vi "Create Instance.vi"() -> (2 "LT_UpgradeFlash":refnum<class "LT_UpgradeFlash.lvclass">)   [LabVIEW 2017, in "LT_UpgradeFlash.lvclass"]
uses:
  LT_UpgradeFlash.lvclass
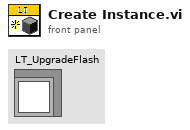
[diagram p1: front panel]
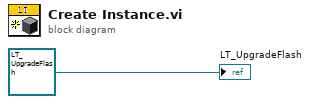
[diagram p0: block diagram]
diagram:
  "LT_UpgradeFlash" <- refnum<class "LT_UpgradeFlash.lvclass"> refnum ("LT_UpgradeFlash.lvclass")
